vi "BundleDataInQueue.vi"(8 "error in (no error)":errorcluster, 11 "DataPacker in":refnum<class "DataPacker.lvclass">) -> (0 "error out":errorcluster, 1 "Enum":T1, 3 "DataPacker out":refnum<class "DataPacker.lvclass">)   [LabVIEW 2018, in "feGEM DataPacker.lvlib"]
uses:
  feGEM DataPacker.lvlib
  StateMachineTypeDef.ctl
  DataPacker.lvclass
  GlobalVariables/DataPacker_Buffer_Usage_Enum.ctl
  GlobalVariables/Set_And_Get_Enum.ctl
panel:
  out "Unique Banks to serialise":i32
  out "Elements bundled for serialisation":i32
  out "DataPacker Queue\nUsage (%)":dbl(knob) scale=0.0..100.0
  out "# elements in queue":i32
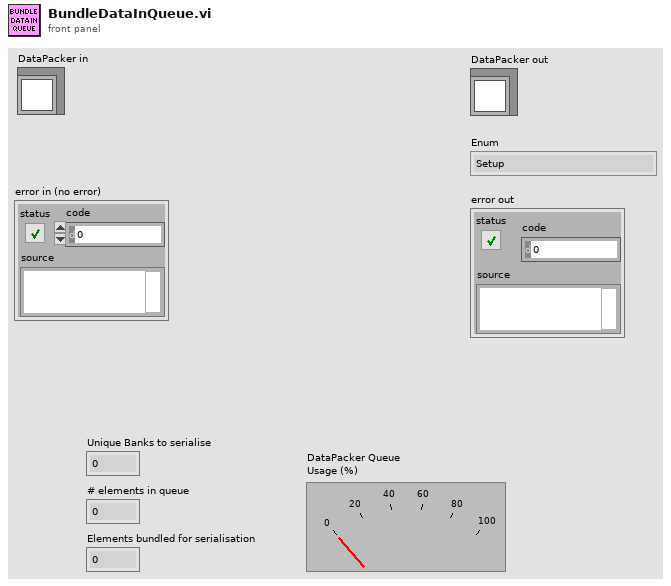
[diagram p1: front panel]
types:
  T1 = typedef "feGEM DataPacker.lvlib/StateMachineTypeDef.ctl" = enum16{"Setup", "Setup SSH", "Connect To Midas", "Get And Set Event Size", "Re-initialise", "Update status", "BundleDataInQueue", "SerializeBundle", "SendData", "Shutdown", "HandleErrorStates", "Wait"}
  T2 = typedef "feGEM DataPacker.lvlib/Set_And_Get_Enum.ctl" = enum16{"Set", "Get"}
  T3 = typedef "feGEM DataPacker.lvlib/DataPacker_Buffer_Usage_Enum.ctl" = enum16{"Get Values", "Set MIDAS Buffer Usage (%)", "Set DataPacker Queue\nUsage (%)"}
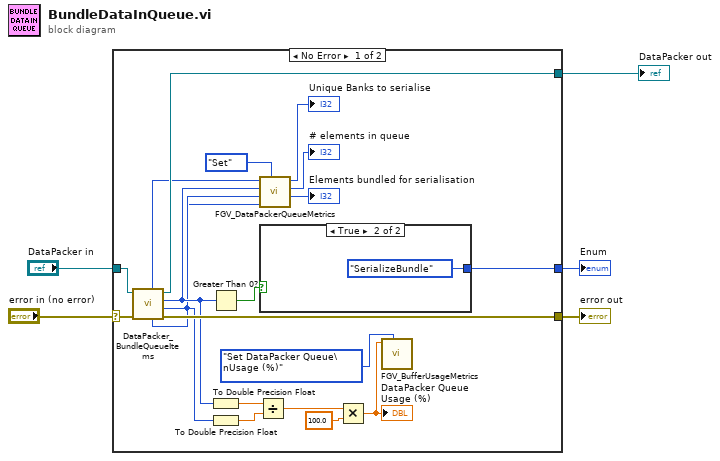
[diagram p0: block diagram]
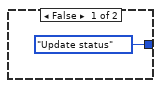
[diagram p2: hidden frame]
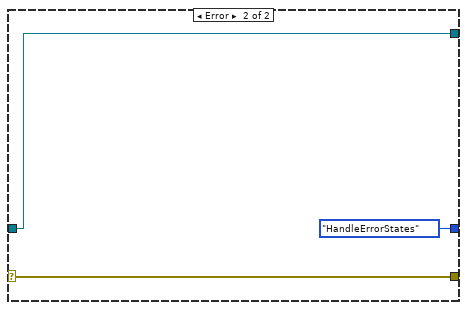
[diagram p3: hidden frame]
diagram:
  n1 = case shown="No Error" "error in (no error)" {
    selector: "error in (no error)" -> [w16 w29]
    tunnel: "DataPacker in" -> [w25 w28]
    tunnel: [w24 w29] -> w2
    tunnel: [w23 w28] -> w3
    tunnel: [w21 StateMachineTypeDef."HandleErrorStates" ("Enum")] -> w4
    frame No Error {
      n2 = call "DataPacker_BundleQueueItems.vi"("error in (no error)"=w16, "DataPacker in"=w25) -> ("error out"=w24:errorcluster, "max queue size"=w6:i32, "# elements in queue"=w11:i32, "DataPacker out"=w23:refnum<class "DataPacker.lvclass">, "Elements bundled for serialisation"=w10:i32, "Unique Banks to serialise"=w12:i32)  [unwired: 4 in]
      n3 = Greater Than 0?(x=w11) -> (x > 0?=w22:bool)
      n4 = To Double Precision Float(number=w11) -> (double precision float=w19:dbl)
      n5 = To Double Precision Float(number=w6) -> (double precision float=w20:dbl)
      n6 = Divide(x=w19, y=w20) -> (x/y=w18:dbl)
      n7 = call "FGV_DataPackerQueueMetrics.vi"("Enum"=Set_And_Get_Enum."Set", "Queue Size"=w6, "Elements bundled for serialisation"=w10, "# elements in queue"=w11, "Unique Banks to serialise"=w12) -> ("Elements bundled for serialisation"=→"Elements bundled for serialisation":i32, "# elements in queue"=→"# elements in queue":i32, "Unique Banks to serialise"=→"Unique Banks to serialise":i32)  [unwired: 3 in, 1 out]
      n8 = case shown="True" w22 {
        tunnel: [StateMachineTypeDef."Update status" ("Enum") StateMachineTypeDef."SerializeBundle" ("Enum")] -> w21
        frame False {
        }
        frame True {
        }
      }
      n9 = Multiply(x=w18, y=100.0) -> (x*y=w15:dbl)
      "DataPacker Queue\nUsage (%)" <- w15
      n10 = call "FGV_BufferUsageMetrics.vi"(7:DataPacker_Buffer_Usage_Enum."Set DataPacker Queue\nUsage (%)", "Input"=w15) -> ()  [unwired: 8 in, 2 out]
    }
    frame Error {
    }
  }
  "Enum" <- w4
  "DataPacker out" <- w3
  "error out" <- w2
